vi "_Center Callee in Caller's BD.vi"(8 "Error In":errorcluster, 10 "Callee VI Refnum (Caller)":refnum<vi>, 11 "Caller VI Refnum (Callee's Caller)":refnum<vi>) -> (0 "Error Out":errorcluster)   [LabVIEW 2017]
doc: "This VI is designed to center a callee VI's window in a caller VI's window.\n\nAuthored by Brandon Steele\nsupport@mooregoodideas.com\nwww.mooregoodideas.com\n\nCopyright (c) 2010, Moore Good Ideas, Inc.\n\nAll rights reserved.\n\nRedistribution and use in source and binary forms, with or without modification, are permitted provided that the following conditions are met:\n\n * Redistributions of source code must retain the above copyright notice, this list of conditions and the following disclaimer.\n * Redistributions in binary form must reproduce the above copyright notice, this list of conditions and the following disclaimer in the documentation and/or other materials provided with the distribution.\n * Neither the name of Moore Good Ideas, Inc. nor the names of its contributors may be used to endorse or promote products derived from this software without specific prior written permission.\n\nTHIS SOFTWARE IS PROVIDED BY THE COPYRIGHT HOLDERS AND CONTRIBUTORS \"AS IS\" AND ANY EXPRESS OR IMPLIED WARRANTIES, INCLUDING, BUT NOT LIMITED TO, THE IMPLIED WARRANTIES OF MERCHANTABILITY AND FITNESS FOR A PARTICULAR PURPOSE ARE DISCLAIMED. IN NO EVENT SHALL THE COPYRIGHT OWNER OR CONTRIBUTORS BE LIABLE FOR ANY DIRECT, INDIRECT, INCIDENTAL, SPECIAL, EXEMPLARY, OR CONSEQUENTIAL DAMAGES (INCLUDING, BUT NOT LIMITED TO, PROCUREMENT OF SUBSTITUTE GOODS OR SERVICES; LOSS OF USE, DATA, OR PROFITS; OR BUSINESS INTERRUPTION) HOWEVER CAUSED AND ON ANY THEORY OF LIABILITY, WHETHER IN CONTRACT, STRICT LIABILITY, OR TORT (INCLUDING NEGLIGENCE OR OTHERWISE) ARISING IN ANY WAY OUT OF THE USE OF THIS SOFTWARE, EVEN IF ADVISED OF THE POSSIBILITY OF SUCH DAMAGE."
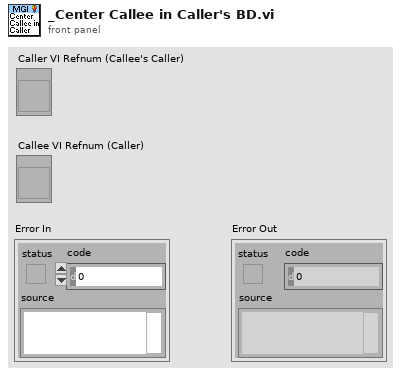
[diagram p1: front panel]
types:
  T1 = typedef "LVRectTypeDef.ctl" = cluster{"Left":i16, "Top":i16, "Right":i16, "Bottom":i16}
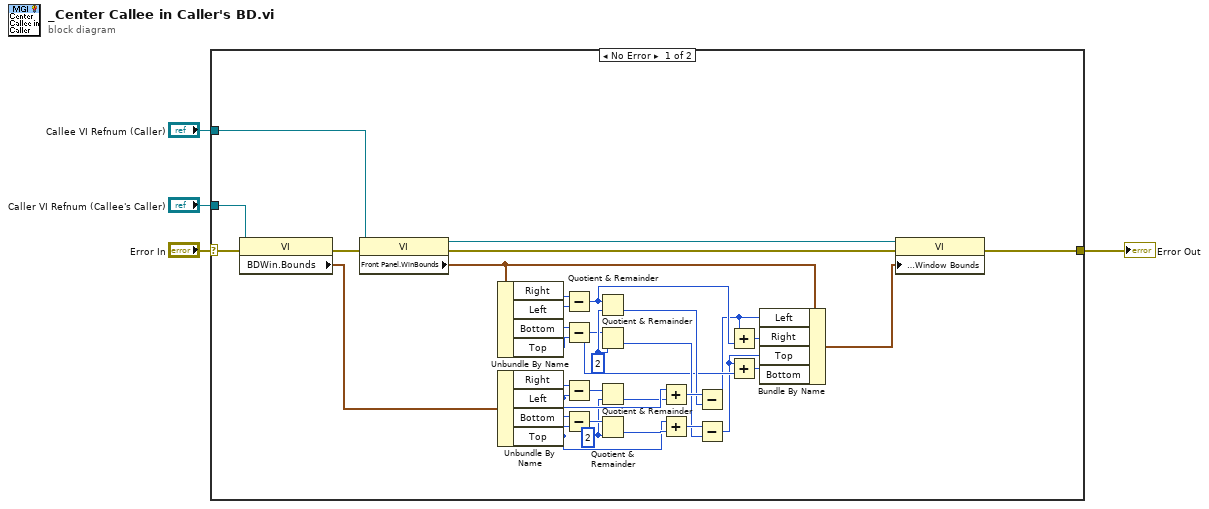
[diagram p0: block diagram]
diagram:
  n1 = case shown="No Error" "Error In" {
    selector: "Error In" -> [w13 w39]
    tunnel: [w38 w39] -> w4
    tunnel: "Caller VI Refnum (Callee's Caller)" -> [w12 _]
    tunnel: "Callee VI Refnum (Caller)" -> [w11 _]
    frame No Error {
      w31 = i16 2 ("y")
      w14 = i16 2 ("y")
      n2 = property class="VI"(reference=w12, error in=w13) -> (error out=w32:errorcluster, "BDWin.Bounds"=w37:T1)  [unwired: 1 out]
      n3 = property class="VI"(reference=w11, error in=w32) -> (reference out=w18:refnum<vi>, error out=w17:errorcluster, "Front Panel.WinBounds"=w6:T1)
      n4 = Unbundle By Name(w6) -> ("Right"=w27:i16, "Left"=w28:i16, "Bottom"=w29:i16, "Top"=w30:i16)
      n5 = Unbundle By Name(w37) -> ("Right"=w36:i16, "Left"=w26:i16, "Bottom"=w35:i16, "Top"=w23:i16)
      n6 = Subtract(x=w27, y=w28) -> (x-y=w16:i16)
      n7 = Subtract(x=w29, y=w30) -> (x-y=w15:i16)
      n8 = Subtract(x=w36, y=w26) -> (x-y=w34:i16)
      n9 = Subtract(x=w35, y=w23) -> (x-y=w33:i16)
      n10 = Quotient & Remainder(x=w16, y=w31) -> (floor(x/y)=w21:i16)  [unwired: 1 out]
      n11 = Quotient & Remainder(x=w15, y=w31) -> (floor(x/y)=w19:i16)  [unwired: 1 out]
      n12 = Quotient & Remainder(x=w34, y=w14) -> (floor(x/y)=w25:i16)  [unwired: 1 out]
      n13 = Quotient & Remainder(x=w33, y=w14) -> (floor(x/y)=w24:i16)  [unwired: 1 out]
      n14 = Add(x=w26, y=w25) -> (x+y=w22:i16)
      n15 = Add(x=w23, y=w24) -> (x+y=w20:i16)
      n16 = Subtract(x=w22, y=w21) -> (x-y=w9:i16)
      n17 = Subtract(x=w20, y=w19) -> (x-y=w8:i16)
      n18 = Add(x=w9, y=w16) -> (x+y=w7:i16)
      n19 = Add(x=w8, y=w15) -> (x+y=w10:i16)
      n20 = Bundle By Name(cluster=w6, "Left"=w9, "Right"=w7, "Top"=w8, "Bottom"=w10) -> (w5:T1)
      n21 = property class="VI"(reference=w18, error in=w17, "Front Panel Window:Window Bounds"=w5) -> (error out=w38:errorcluster)  [unwired: 1 out]
    }
    frame Error {
    }
  }
  "Error Out" <- w4
